vi "peakFinding example.vi"() -> ()   [LabVIEW 2018]
uses:
  <vilib>/Utility/miscctls.llb/LVAnnotationListTypeDef.ctl
  Editor/ctl/editScriptState.ctl
panel:
  in  "runBtn":bool
  in  "editorBtn":bool
  in  "error in (no error)":errorcluster
  in  "ampTh":dbl=-inf
  in  "slopeTh":dbl=-inf
  in  "window":dbl=100.0 format="%#_13g"
  in  "dt":dbl=1.0 format="%#_13g"
  out "peakFinding":cluster{"xData":dbl[], "yData":sgl[]}[](graph)
  out "rawData":cluster{"xData":dbl[], "noise":sgl[]}(graph)
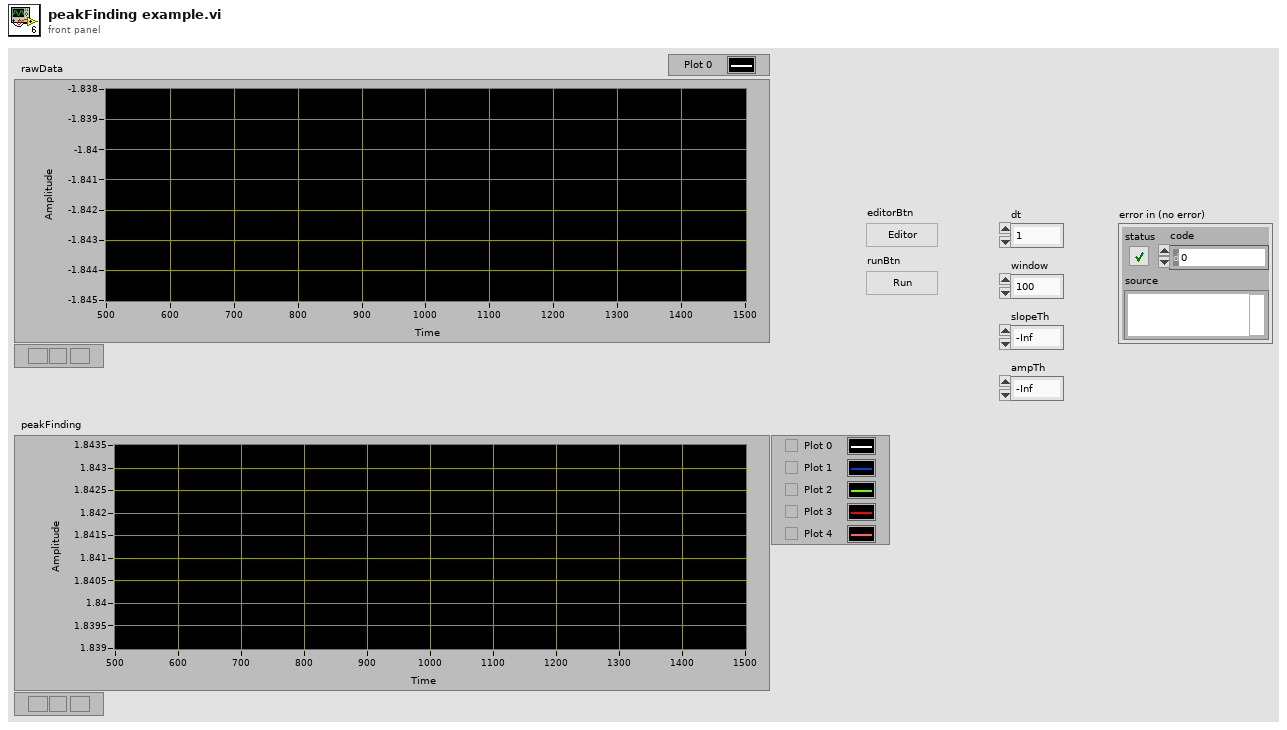
[diagram p1: front panel]
types:
  T1 = typedef "editScriptState.ctl" = enum16{"init", "loadScript", "newScript", "runScript", "close"}
  T2 = typedef "LVAnnotationListTypeDef.ctl" = cluster{"Name":string, "Color":u32, "Style":u8, "Point Style":u8, "Name Visible":bool, "Allow Drag":bool, "Annotation Mode":u32, "Plot":i32, "Index":i32, "Position":cluster{"X":dbl, "Y":dbl}, "X Scale":u32, "Y Scale":u32, "Show Arrow":bool, "Lock Name":bool, "Plot Area":i32, "Label Offset":cluster{"X":dbl, "Y":dbl}}[]
  T3 = cluster{"Name":string, "Color":i32, "Style":u8, "Point Style":i32, "Name Visible":bool, "Allow Drag":bool, "Annotation Mode":u32, "Plot":i32, "Index":i32, "Position":cluster{"X":dbl, "Y":dbl}, "X Scale":u32, "Y Scale":u32, "Show Arrow":bool, "Lock Name":bool, "Plot Area":i32, "Label Offset":cluster{"X":dbl, "Y":dbl}}[]
  T4 = cluster{"priDt":dbl, "priXData":dbl[], "priYData":sgl[], "beta":dbl[]}
  T5 = cluster{"startTime":dbl, "scanSig":cluster{"priDt":dbl, "priXData":dbl[], "priYData":sgl[], "beta":dbl[]}[]}
  T6 = cluster{"priDt":dbl, "priXData":dbl[], "priYData":sgl[], "beta":dbl[]}[]
  T7 = cluster{"startTime":dbl, "scanData":cluster{"dt":dbl, "xdata":dbl[], "ydata":sgl[], "beta":dbl[]}[], "xyXLabel":string, "xyYLabel":string, "peakData":cluster{"xLeftIdx":u32[], "xCenterIdx":u32[], "xRightIdx":u32[], "baseline":sgl[], "halfHeight":dbl[]}[]}
  T8 = cluster{"dt":dbl, "xdata":dbl[], "ydata":sgl[], "beta":dbl[]}[]
  T9 = cluster{"xLeftIdx":u32[], "xCenterIdx":u32[], "xRightIdx":u32[], "baseline":sgl[], "halfHeight":dbl[]}[]
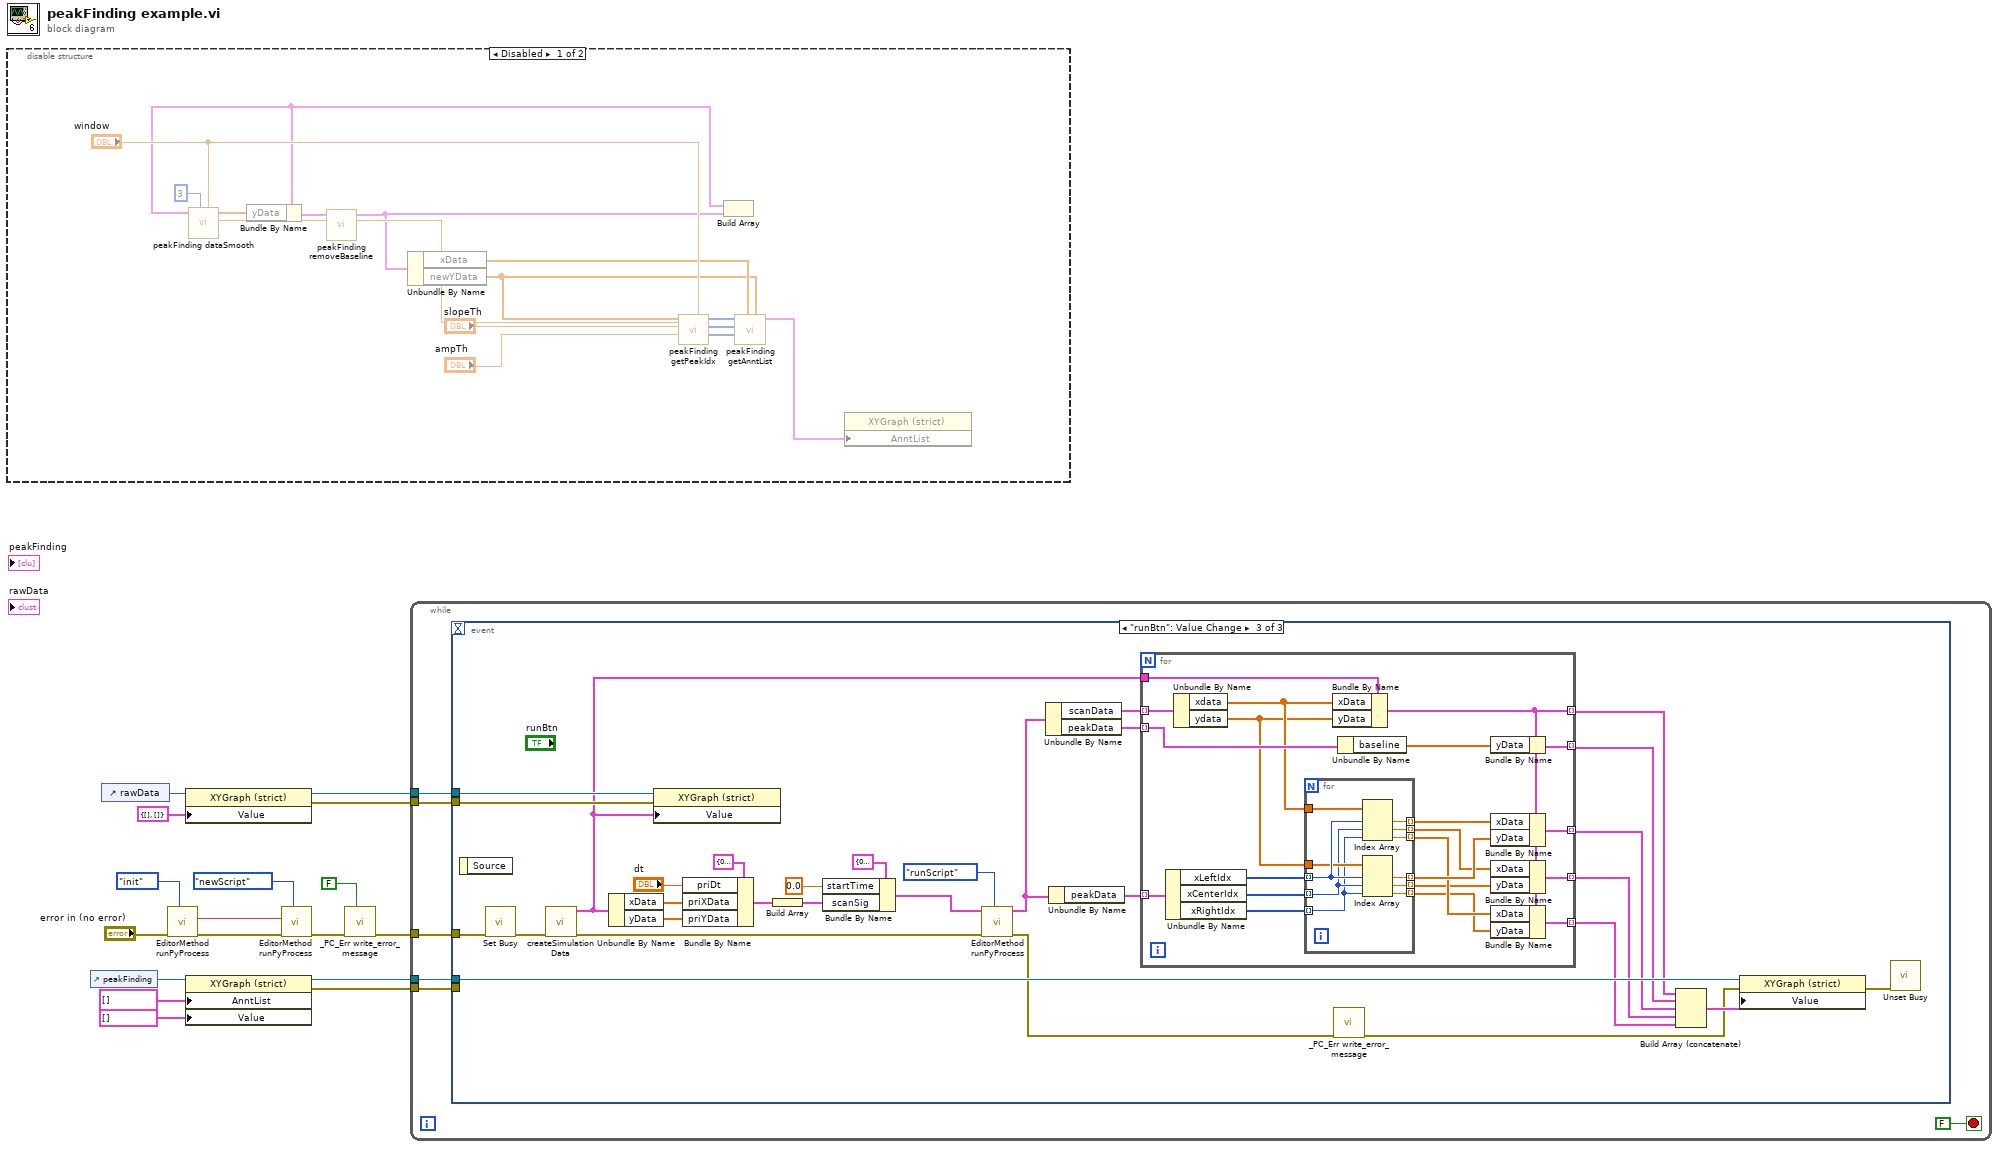
[diagram p0: block diagram]
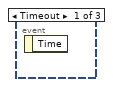
[diagram p3: hidden frame]
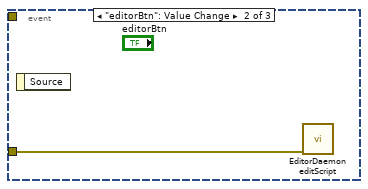
[diagram p4: hidden frame]
diagram:
  n1 = disable-structure shown="Disabled" {
    frame Disabled {
      n2 = call "peakFinding dataSmooth.vi"("Window"="window", "Type"=u8 3) -> ("yData"=w24:dbl[], "dt"=w30:dbl, "rawData"=w19:cluster{"xData":dbl[], "yData":dbl[]})  [unwired: 7 in]
      n3 = Bundle By Name(cluster=w19, "yData"=w24) -> (w23:cluster{})
      n4 = call "peakFinding removeBaseline.vi"("sourceData"=w23) -> ("signalData"=w20:cluster{"xData":dbl[], "newYData":dbl[]})  [unwired: 8 in, 2 out]
      n5 = Unbundle By Name(w20) -> ("xData"=w22:dbl[], "newYData"=w21:dbl[])
      n6 = call "peakFinding getPeakIdx.vi"("window"="window", "dt"=w30, "ampTh"="ampTh", "slopeTh"="slopeTh", "yData"=w21) -> ("rightIdx"=w25:i32[], "leftIdx"=w26:i32[], "peakIdx"=w27:i32[])  [unwired: 4 in]
      n7 = Build Array(w19, w20) -> ()  [unwired: 1 out]
      n8 = call "peakFinding getAnntList.vi"("1stDiffData"=w21, "xData"=w22, "rightIdx"=w25, "leftIdx"=w26, "peakIdx"=w27) -> ("anntList"=w18:T3)  [unwired: 6 in]
      n9 = property class="XYGraph (strict)"("AnntList"=w18) -> ()  [unwired: 2 in, 2 out]
    }
    frame Enabled {
    }
  }
  n10 = control-ref of="peakFinding"() -> (w14:refnum<vi>)
  n11 = control-ref of="rawData"() -> (w9:refnum<vi>)
  n12 = call "EditorMethod runPyProcess.vi"("func"=editScriptState."init", "error in (no error)"="error in (no error)") -> ("error out"=w17:errorcluster, "pyCode"=w16:string)  [unwired: 6 in, 2 out]
  n13 = property class="XYGraph (strict)"(reference=w9, "Value"=cluster{"xData":dbl[], "noise":sgl[]} {"xData"=[], "noise"=[]}) -> (reference out=w7:refnum<vi>, error out=w6:errorcluster)  [unwired: 1 in]
  n14 = property class="XYGraph (strict)"(reference=w14, "AnntList"=T2 [] ("Annotation List"), "Value"=cluster{"xData":dbl[], "yData":sgl[]}[] []) -> (reference out=w11:refnum<vi>, error out=w12:errorcluster)  [unwired: 1 in]
  n15 = call "EditorMethod runPyProcess.vi"("func"=editScriptState."newScript", "error in (no error)"=w17, "newScriptCode"=w16) -> ("error out"=w5:errorcluster)  [unwired: 5 in, 3 out]
  n16 = call "_PC_Err write_error_message.vi"("show msg( T )"=FALSE, "error in"=w5) -> ("error out"=w4:errorcluster)  [unwired: 9 in]
  n17 = while {
    tunnel: w4 -> [w38]
    tunnel: w12 -> [w36]
    tunnel: w11 -> [w35]
    tunnel: w7 -> [w34]
    tunnel: w6 -> [w33]
    stop <- FALSE stop-if-true
    n18 = event shown="[2] \"runBtn\": Value Change" {
      selector: _ -> [_ _ _]
      dyn-events: _ -> [_ _ _]
      timeout: _ -> [_ _ _]
      tunnel: w38 -> [_ w39 w51]
      tunnel: w36 -> [_ _ _]
      tunnel: w35 -> [_ _ w61]
      tunnel: w34 -> [_ _ w60]
      tunnel: w33 -> [_ _ w59]
      event Timeout {
        n19 = event-data() -> ()  [unwired: 1 in, 1 out]
      }
      event "editorBtn": Value Change {
        n20 = event-data() -> ()  [unwired: 1 in, 1 out]
        n21 = call "EditorDaemon editScript.vi"("error in (no error)"=w39) -> ()  [unwired: 10 in, 1 out]
      }
      event "runBtn": Value Change {
        n22 = event-data() -> ()  [unwired: 1 in, 1 out]
        n23 = call <vilib>:"Set Busy.vi"("error in (no error)"=w51) -> ("error out"=w50:errorcluster)  [unwired: 9 in, 1 out]
        n24 = call "createSimulationData.vi"("error in (no error)"=w50) -> ("error out"=w69:errorcluster, "rawData"=w58:cluster{"xData":dbl[], "yData":sgl[]})  [unwired: 9 in]
        n25 = Unbundle By Name(w58) -> ("xData"=w66:dbl[], "yData"=w65:sgl[])
        n26 = property class="XYGraph (strict)"(reference=w60, error in=w59, "Value"=w58) -> ()  [unwired: 2 out]
        n27 = Bundle By Name(cluster=T4 {"priDt"=0.0, "priXData"=[], "priYData"=[], "beta"=[]} ("ScanSigSec"), "priDt"="dt", "priXData"=w66, "priYData"=w65) -> (w56:T4)
        n28 = Build Array(w56) -> (w63:T6)
        n29 = Bundle By Name(cluster=T5 {"startTime"=0.0, "scanSig"=[]} ("dataParam"), "startTime"=0.0, "scanSig"=w63) -> (w41:T5)
        n30 = call "EditorMethod runPyProcess.vi"("func"=editScriptState."runScript", "error in (no error)"=w69, "dataParam"=w41) -> ("error out"=w49:errorcluster, "newSigInfo"=w46:T7)  [unwired: 5 in, 2 out]
        n31 = Unbundle By Name(w46) -> ("scanData"=w57:T8, "peakData"=w55:T9)
        n32 = Unbundle By Name(w46) -> ("peakData"=w45:T9)
        n33 = for {
          tunnel: w58 -> [w90]
          tunnel: w57 -> [w89] mode=indexing
          tunnel: [w74] -> w54 mode=indexing
          tunnel: w55 -> [w88] mode=indexing
          tunnel: [w85] -> w53 mode=indexing
          tunnel: w45 -> [w86] mode=indexing
          tunnel: [w84] -> w44 mode=indexing
          tunnel: [w75] -> w43 mode=indexing
          tunnel: [w73] -> w42 mode=indexing
          n34 = Unbundle By Name(w86) -> ("xLeftIdx"=w72:u32[], "xCenterIdx"=w71:u32[], "xRightIdx"=w70:u32[])
          n35 = Unbundle By Name(w89) -> ("xdata"=w83:dbl[], "ydata"=w82:sgl[])
          n36 = for {
            tunnel: w72 -> [w101] mode=indexing
            tunnel: w83 -> [w100]
            tunnel: w82 -> [w99]
            tunnel: [w98] -> w80 mode=indexing
            tunnel: [w97] -> w81 mode=indexing
            tunnel: w71 -> [w96] mode=indexing
            tunnel: w70 -> [w95] mode=indexing
            tunnel: [w94] -> w79 mode=indexing
            tunnel: [w93] -> w78 mode=indexing
            tunnel: [w92] -> w77 mode=indexing
            tunnel: [w91] -> w76 mode=indexing
            n37 = Index Array(array=w100, index #1=w101, index #2=w96, index #3=w95) -> (element #1=w97:dbl, element #2=w94:dbl, element #3=w93:dbl)
            n38 = Index Array(array=w99, index #1=w101, index #2=w96, index #3=w95) -> (element #1=w98:sgl, element #2=w92:sgl, element #3=w91:sgl)
          }
          n39 = Bundle By Name(cluster=w90, "xData"=w83, "yData"=w82) -> (w74:cluster{"xData":dbl[], "yData":sgl[]})
          n40 = Unbundle By Name(w88) -> ("baseline"=w87:sgl[])
          n41 = Bundle By Name(cluster=w74, "yData"=w87) -> (w85:cluster{"xData":dbl[], "yData":sgl[]})
          n42 = Bundle By Name(cluster=w74, "xData"=w81, "yData"=w80) -> (w84:cluster{"xData":dbl[], "yData":sgl[]})
          n43 = Bundle By Name(cluster=w74, "xData"=w79, "yData"=w77) -> (w75:cluster{"xData":dbl[], "yData":sgl[]})
          n44 = Bundle By Name(cluster=w74, "xData"=w78, "yData"=w76) -> (w73:cluster{"xData":dbl[], "yData":sgl[]})
        }
        n45 = call "_PC_Err write_error_message.vi"("error in"=w49) -> ("error out"=w48:errorcluster)  [unwired: 10 in]
        n46 = Build Array (concatenate)(w54, w53, w44, w43, w42) -> (w52:cluster{"xData":dbl[], "yData":sgl[]}[])
        n47 = property class="XYGraph (strict)"(reference=w61, error in=w48, "Value"=w52) -> (error out=w47:errorcluster)  [unwired: 1 out]
        n48 = call <vilib>:"Unset Busy.vi"("error in (no error)"=w47) -> ()  [unwired: 10 in, 1 out]
      }
    }
  }
